vi "1775E_Login List.vi"(8 "error in (no error)":errorcluster, 11 "data":variant[][](array[variant])) -> (0 "error out":errorcluster)   [LabVIEW 2020]
uses:
  <vilib>/Utility/miscctls.llb/LVRowAndColumnUnsignedTypeDef.ctl
panel:
  in  "Exit":bool
  in  "User list":i32(listbox)
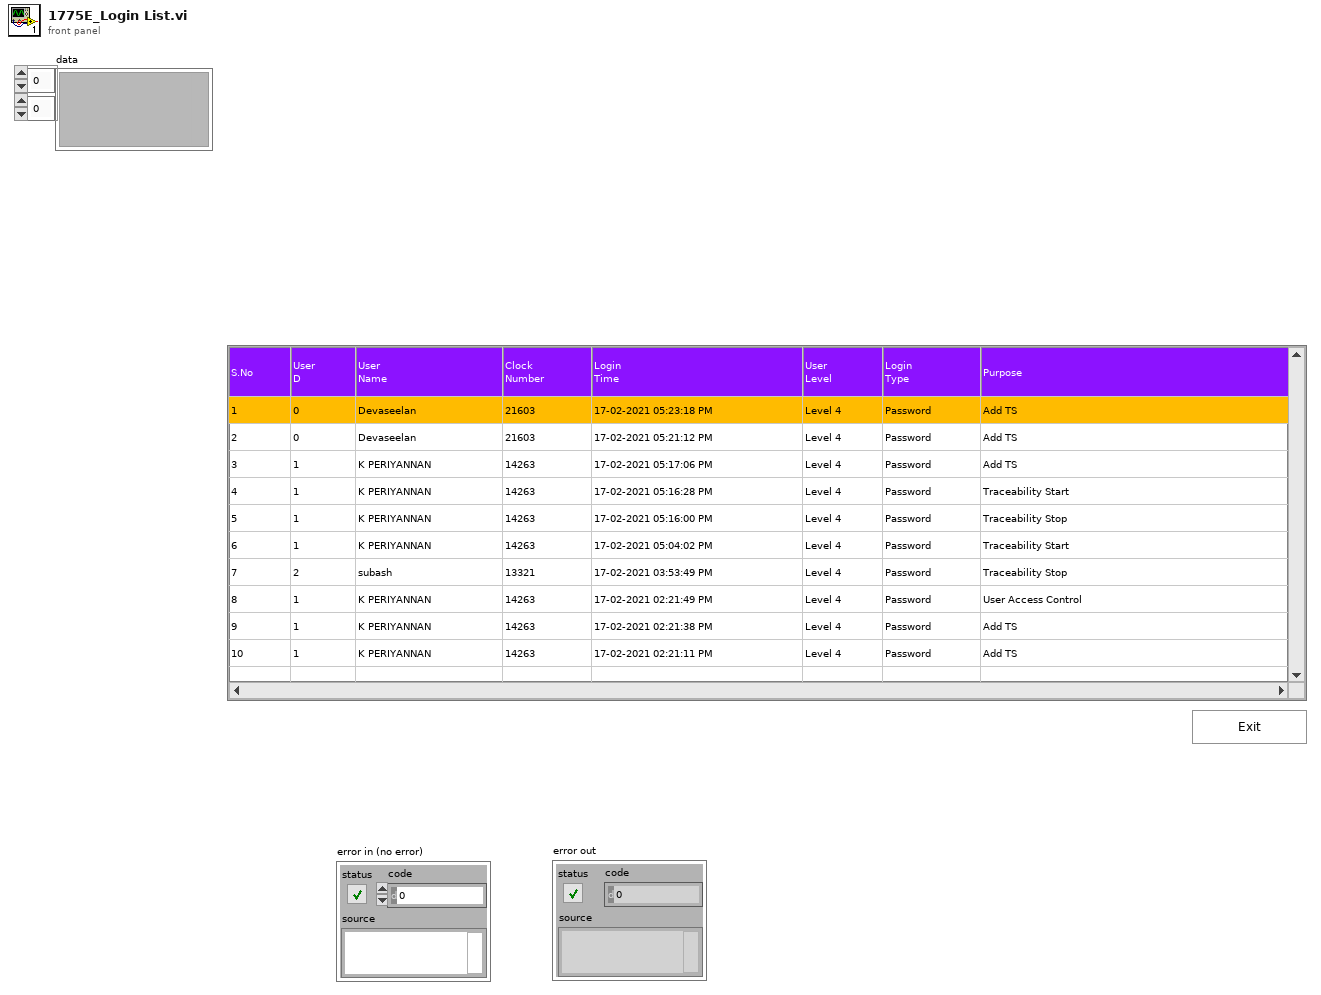
[diagram p1: front panel]
types:
  T1 = typedef "LVRowAndColumnUnsignedTypeDef.ctl" = cluster{"Row":u32, "Column":u32}
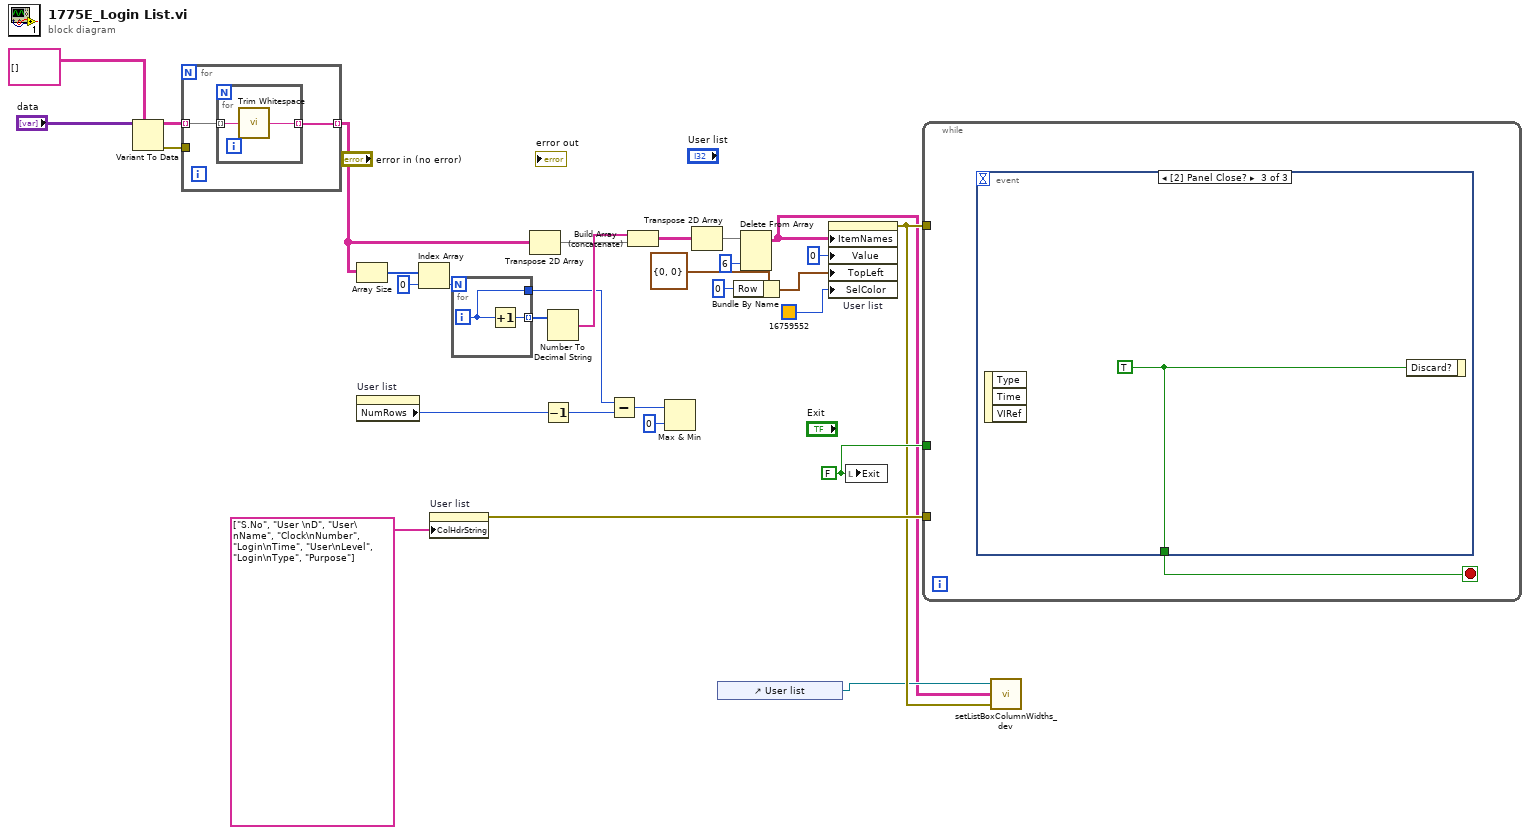
[diagram p0: block diagram]
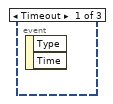
[diagram p2: hidden frame]
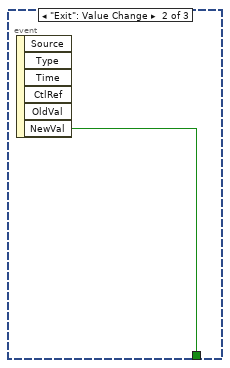
[diagram p3: hidden frame]
diagram:
  w21 = FALSE ("Exit")
  n1 = Variant To Data(type=string[][] [] ("Array"), Variant="data") -> (data=w20:string[][], error out=w18:errorcluster)  [unwired: 1 in]
  n2 = for {
    tunnel: w20 -> [w32] mode=indexing
    tunnel: [w31] -> w19 mode=indexing
    tunnel: w18 -> [_]
    n3 = for {
      tunnel: w32 -> [w34] mode=indexing
      tunnel: [w33] -> w31 mode=indexing
      n4 = call <vilib>:"Trim Whitespace.vi"("string"=w34) -> ("trimmed string"=w33:string)  [unwired: 1 in]
    }
  }
  n5 = Array Size(array=w19) -> (size(s)=w28:i32[])
  n6 = property on="User list" class="MCListbox (strict)"() -> ("NumRows"=w14:u32)  [unwired: 2 in, 2 out]
  n7 = Index Array(array=w28, index=0) -> (element=w26:i32)
  n8 = property on="User list" class="MCListbox (strict)"("ColHdrString"=string[] ["S.No", "User \nD", "User\nName", "Clock\nNumber", "Login\nTime", "User\nLevel", "Login\nType", "Purpose"] ("Column Header Strings[]")) -> (error out=w16:errorcluster)  [unwired: 2 in, 1 out]
  n9 = for {
    N: w26 -> [_]
    tunnel: [w36] -> w25 mode=indexing
    tunnel: [w35] -> w15
    i -> [w35]
    n10 = Increment(x=w35) -> (x+1=w36:i32)
  }
  n11 = Transpose 2D Array(2D array=w19) -> (transposed array=w22:string[][])
  n12 = Decrement(x=w14) -> (x-1=w10:u32)
  n13 = Number To Decimal String(number=w25) -> (decimal integer string=w23:string[])  [unwired: 1 in]
  n14 = Subtract(x=w15, y=w10) -> (x-y=w13:u32)
  n15 = Build Array (concatenate)(w23, w22) -> (w24:string[][])
  n16 = Max & Min(x=w13, y=u32 0) -> ()  [unwired: 2 out]
  n17 = Transpose 2D Array(2D array=w24) -> (transposed array=w5:string[][])
  n18 = control-ref of="User list"() -> (w7:refnum<vi>)
  n19 = Bundle By Name(cluster=T1 {"Row"=0, "Column"=0} ("Top Left Visible Cell"), "Row"=u32 0) -> (w6:T1)
  n20 = Delete From Array(array=w5, index (col)=6 ("disabled index (col)")) -> (array with subset deleted=w3:string[][])  [unwired: 2 in, 1 out]
  n21 = property on="User list" class="MCListbox (strict)"("ItemNames"=w3, "Value"=0 ("User list"), "TopLeft"=w6, "SelColor"=u32 16759552 ("Selection Color")) -> (error out=w8:errorcluster)  [unwired: 2 in, 1 out]
  n22 = local write "Exit"(w21) -> ()
  n23 = while {
    tunnel: w21 -> [_]
    tunnel: w8 -> [_]
    tunnel: w16 -> [_]
    stop <- w37 stop-if-true
    n24 = event shown="[2] Panel Close?" {
      selector: _ -> [_ _ _]
      dyn-events: _ -> [_ _ _]
      timeout: _ -> [_ _ _]
      tunnel: [_ w38 w39] -> w37
      event Timeout {
        n25 = event-data() -> ()  [unwired: 1 in, 2 out]
      }
      event "Exit": Value Change {
        n26 = event-data() -> ("NewVal"=w38:bool)  [unwired: 1 in, 5 out]
      }
      event Panel Close? {
        w39 = TRUE ("Discard?")
        n27 = event-data() -> ()  [unwired: 1 in, 3 out]
        n28 = event-data("Discard?"=w39) -> ()  [unwired: 1 in, 1 out]
      }
    }
  }
  n29 = call "setListBoxColumnWidths_dev.vi"("error in (no error)"=w8, "table data"=w3, "MCListbox Refnum"=w7) -> ()
